vi "Write Variant (dyn).vi"(10 "Variant":variant, 11 "Test Object in":refnum<class "Test Object.lvclass">) -> (3 "Test Object out":refnum<class "Test Object.lvclass">)   [LabVIEW 2015, in "Test Object.lvclass"]
uses:
  Test Object.lvclass
  Test Object.lvclass/Test Object.ctl
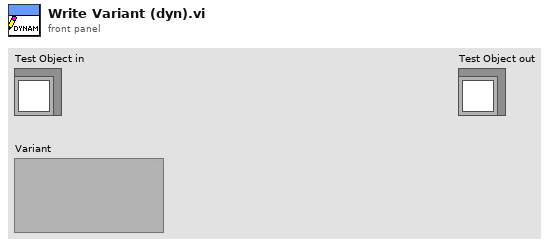
[diagram p1: front panel]
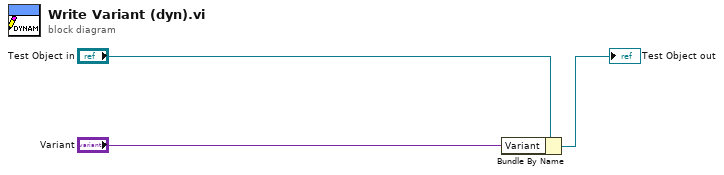
[diagram p0: block diagram]
diagram:
  n1 = Bundle By Name(cluster="Test Object in", "Variant"="Variant") -> (→"Test Object out":refnum<class "Test Object.lvclass">)
